vi "LaserFinding_Lines_v6.vi"(0 "Image In":T2, 7 "error in":errorcluster) -> (20 "Image Out":T2, 21 "Straight Edge (Find Vert. Edge)":T1 {"Point2 (Real-World)"."Y" format="%.2f"; "Point2 (Real-World)"."X" format="%.2f"; "Point1 (Real-World)"."Y" format="%.2f"; "Point1 (Real-World)"."X" format="%.2f"; "Point2 (Pixels)"."Y" format="%.2f"; "Point2 (Pixels)"."X" format="%.2f"; "Point1 (Pixels)"."Y" format="%.2f"; "Point1 (Pixels)"."X" format="%.2f"}, 22 "Straight Edge (Find Horiz. Edge)":T1 {"Point2 (Real-World)"."Y" format="%.2f"; "Point2 (Real-World)"."X" format="%.2f"; "Point1 (Real-World)"."Y" format="%.2f"; "Point1 (Real-World)"."X" format="%.2f"; "Point2 (Pixels)"."Y" format="%.2f"; "Point2 (Pixels)"."X" format="%.2f"; "Point1 (Pixels)"."Y" format="%.2f"; "Point1 (Pixels)"."X" format="%.2f"}, 27 "error out":errorcluster)   [LabVIEW 2014]
uses:
  <vilib>/vision/Image Controls.llb/IMAQ Image.ctl
  <vilib>/vision/Measure.llb/Edge Options.ctl
  <vilib>/vision/Measure.llb/Edge Polarity.ctl
  <vilib>/vision/Measure.llb/Straight Edge Options.ctl
  <vilib>/vision/Measure.llb/Straight Edge Process.ctl
  <vilib>/vision/NI_Vision_Development_Module.lvlib
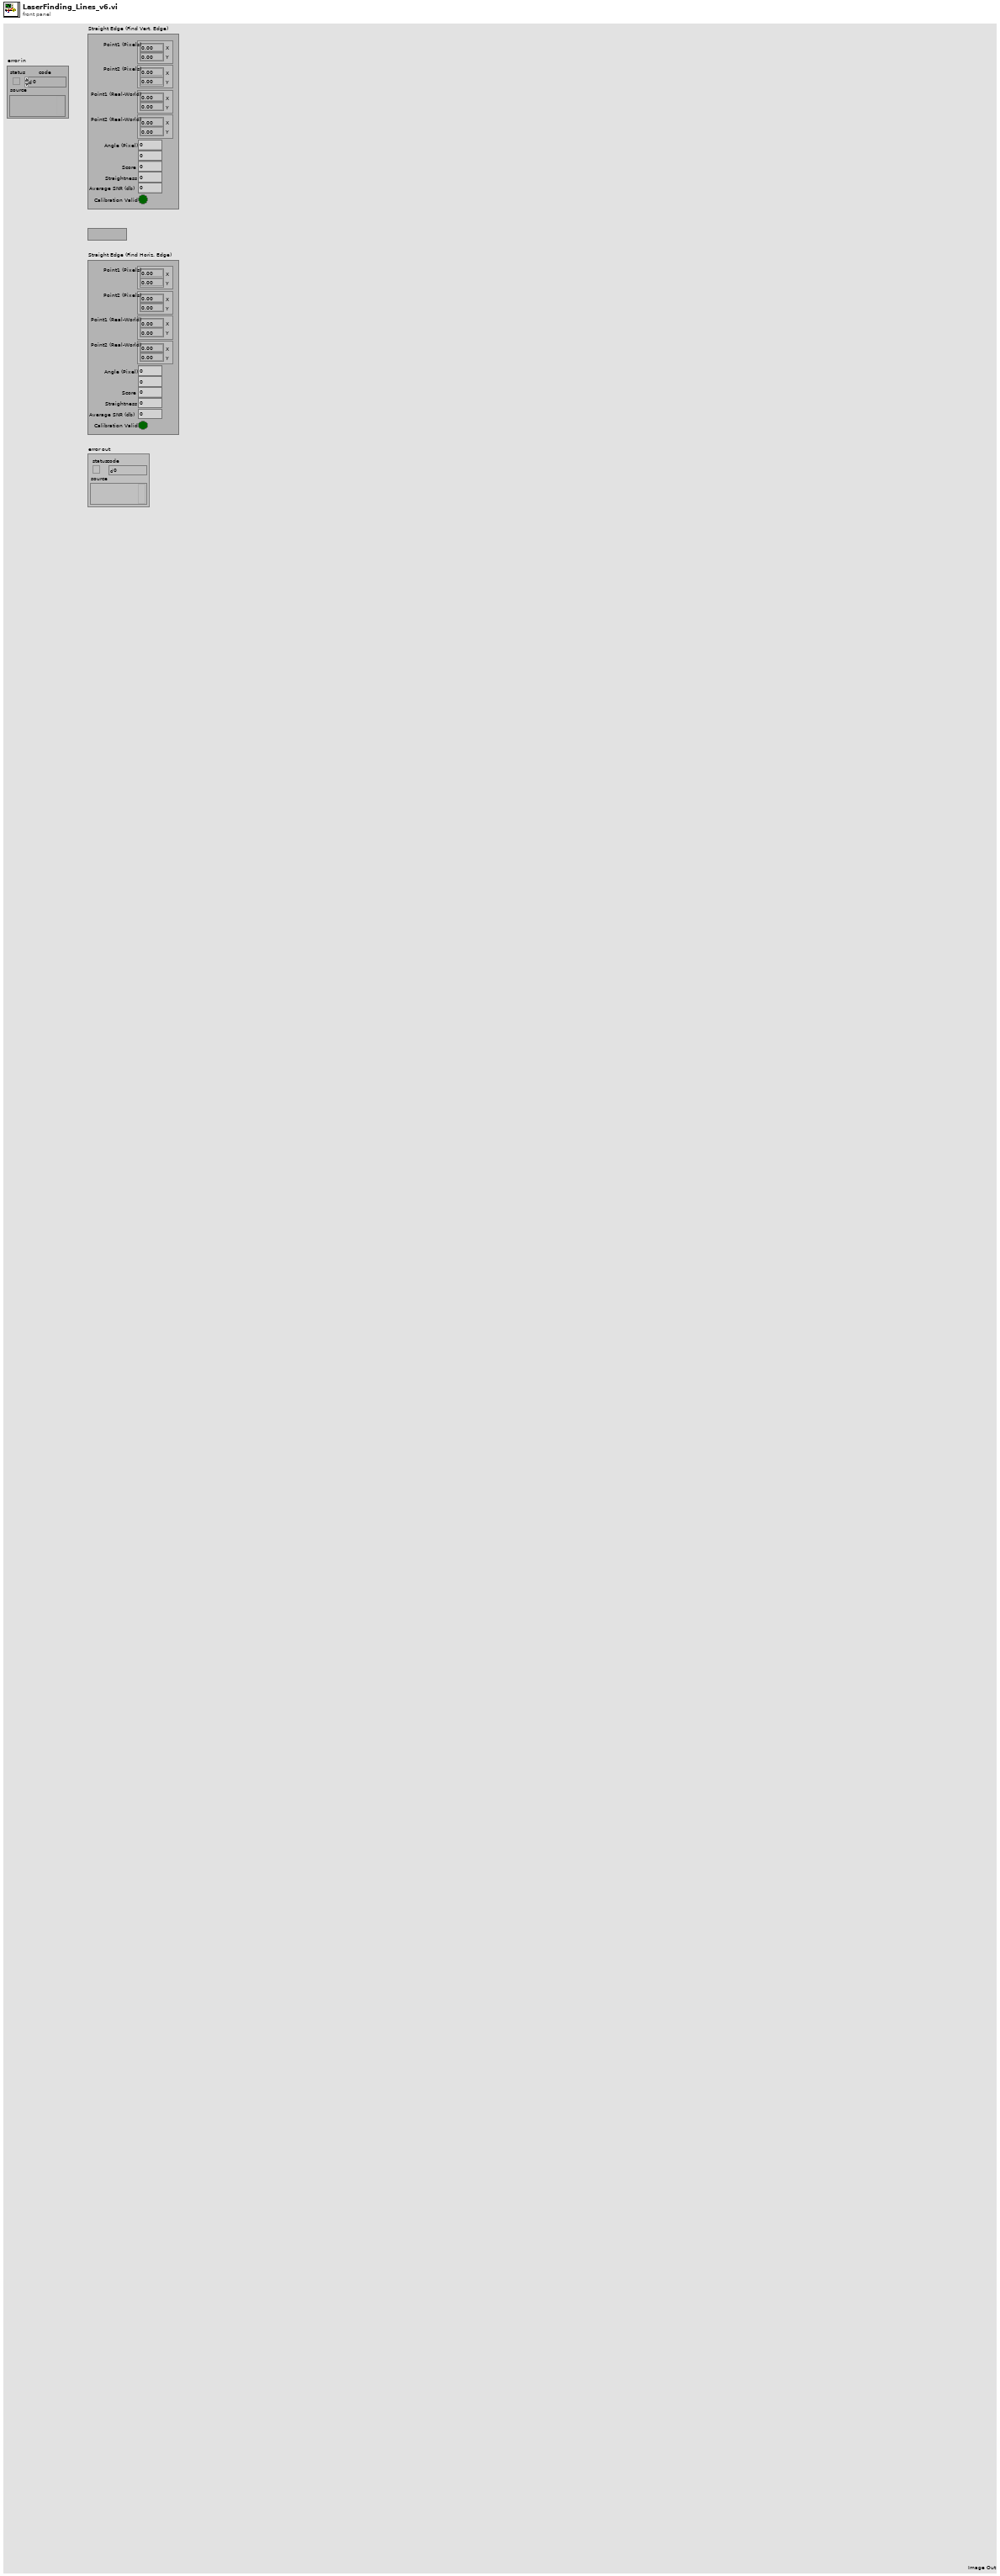
[diagram p1: front panel]
types:
  T1 = cluster{"Point1 (Pixels)":cluster{"X":sgl, "Y":sgl}, "Point2 (Pixels)":cluster{"X":sgl, "Y":sgl}, "Point1 (Real-World)":cluster{"X":sgl, "Y":sgl}, "Point2 (Real-World)":cluster{"X":sgl, "Y":sgl}, "Angle (Pixel)":dbl, "Angle (Real-World)":dbl, "Score":dbl, "Straightness":dbl, "Average SNR (db)":dbl, "Calibration Valid":bool}
  T2 = typedef "IMAQ Image.ctl" = refnum<image>
  T3 = typedef "Edge Options.ctl" = cluster{"Edge Polarity":T4, "Kernel Size":u32, "Width":u32, "Minimum Edge Strength":sgl, "Interpolation Type":enum32{"Zero Order", "Bilinear", "Quadratic", "Cubic", "Bilinear Fixed"}, "Data Processing Method":enum32{"Average", "Median"}}
  T4 = typedef "Edge Polarity.ctl" = u32
  T5 = cluster{"Search Direction":u32, "Edge Options":T3, "Show Search Area":bool, "Show Search Lines":bool, "Show Edges Found":bool, "Show Result":bool, "Search Area Color":u32, "Search Lines Color":u32, "Edge Locations Color":u32, "Result Color":u32, "Overlay Group Name":string}
  T6 = typedef "Straight Edge Options.ctl" = cluster{"Number of Lines":i32, "Type":T7, "Min. Score":dbl, "Max. Score":dbl, "Orientation":dbl, "Angle Range":dbl, "Angle Tolerance":dbl, "Step Size":u32, "Min. SNR (db)":dbl, "Min. Points (%)":dbl, "Hough Iterations":i32}
  T7 = typedef "Straight Edge Process.ctl" = enum32{"First Edge Rake", "Best Edge Rake", "Hough Edge Rake", "First Edge Projection", "Best Edge Projection"}
  T8 = cluster{"Global Rectangle":i32[], "Contours":cluster{"ID":enum32{"External", "Internal"}, "Type":u32, "Coordinates":i32[]}[]}
  T9 = cluster{"Measurement Parameter":i32, "Range Lower Value":dbl, "Range Upper Value":dbl, "Range":bool, "Measurement Type":bool}[]
  T10 = typedef "Image Type" = u32
  T11 = cluster{"histogram":u32[], "Minimal Value":sgl, "Maximal Value":sgl, "Starting Value":sgl, "Interval Width":sgl, "Mean Value":sgl, "Standard  Variation":sgl, "Area (pixels)":i32}
  T12 = cluster{"Point1 (Pixels)":cluster{"X":sgl, "Y":sgl}, "Point2 (Pixels)":cluster{"X":sgl, "Y":sgl}, "Point1 (Real-World)":cluster{"X":sgl, "Y":sgl}, "Point2 (Real-World)":cluster{"X":sgl, "Y":sgl}, "Angle (Pixel)":dbl, "Angle (Real-World)":dbl, "Score":dbl, "Straightness":dbl, "Average SNR (db)":dbl, "Calibration Valid":bool}[]
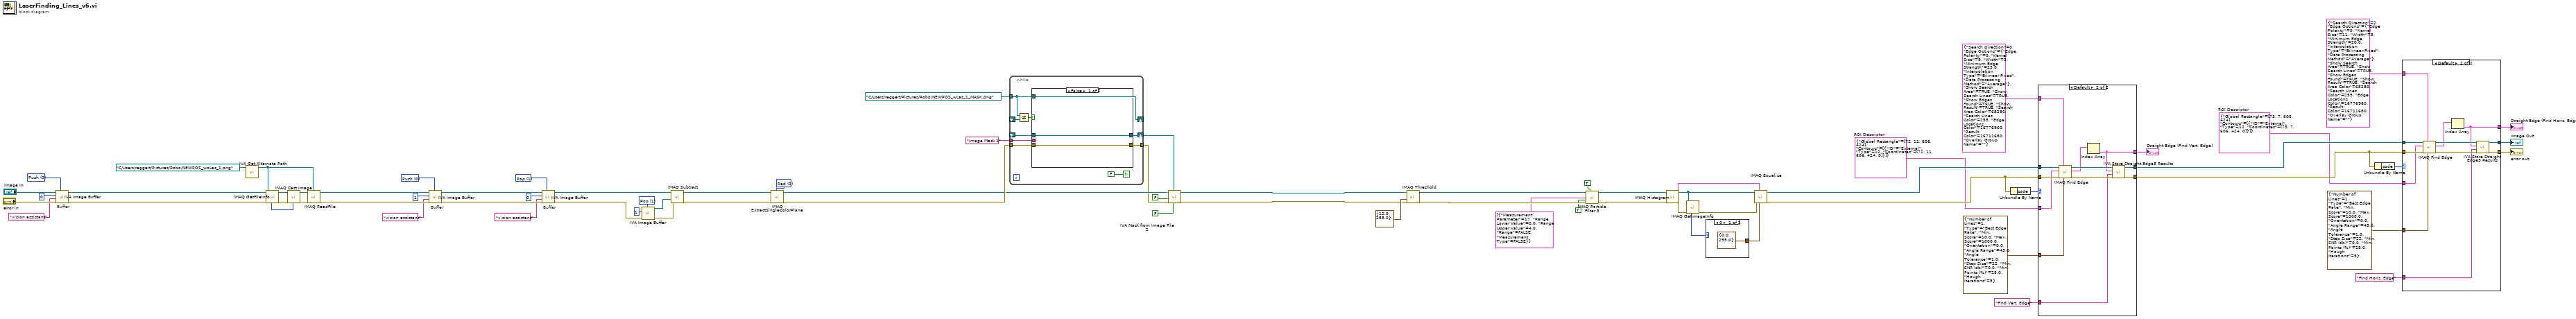
[diagram p0: block diagram]
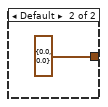
[diagram p4: hidden frame]
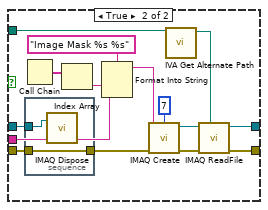
[diagram p5: hidden frame]
diagram:
  w10 = T8 {"Global Rectangle"=[73, 7, 606, 424], "Contours"=[{"ID"=enum."External", "Type"=12, "Coordinates"=[73, 7, 606, 424, 0]}]}  # ROI Descriptor
  w18 = T8 {"Global Rectangle"=[72, 11, 606, 424], "Contours"=[{"ID"=enum."External", "Type"=12, "Coordinates"=[72, 11, 606, 424, 0]}]}  # ROI Descriptor
  w43 = 0 items=["Red", "Green", "Blue", "Hue", "Saturation", "Luminance", "Value", "Intensity"] ("Color Plane")
  w49 = u16 1 items=["Push", "Pop", "Reset"] ("Function")
  w52 = u16 1 items=["Push", "Pop", "Reset"] ("Function")
  w57 = u16 0 items=["Push", "Pop", "Reset"] ("Function")
  w70 = u16 0 items=["Push", "Pop", "Reset"] ("Function")
  # "Buffer"
  # "Buffer"
  # "Buffer"
  n1 = call <vilib>:"IVA Image Buffer.vi"("Function"=w70, "error in (no error)"="error in", "Prefix"="vision assistant", "Buffer #"=0, "Image In"="Image In") -> ("error out"=w71:errorcluster, "Image Out"=w64:T2)  [unwired: 5 out]
  n2 = call <vilib>:"IVA Get Alternate Path.vi"("Path In"=path "C:/Users/reggert/Pictures/Robo/NEWPOS_woLas_1.png" ("File Path")) -> ("Path Out"=w60:path)  [unwired: 10 out]
  n3 = call "IMAQ GetFileInfo"("error in (no error)"=w71, "File Path"=w60) -> ("error out"=w66:errorcluster, "Image Type"=w62:T10)  [unwired: 8 out]
  n4 = call "IMAQ Cast Image"("Image Type"=w62, "error in (no error)"=w66, "Image Src"=w64) -> ("error out"=w65:errorcluster, "Image Dst Out"=w63:T2)  [unwired: 3 in, 4 out]
  n5 = call "IMAQ ReadFile"("File Path"=w60, "error in (no error)"=w65, "Image"=w63) -> ("error out"=w67:errorcluster, "Image Out"=w59:T2)  [unwired: 2 in, 5 out]
  n6 = call <vilib>:"IVA Image Buffer.vi"("Function"=w57, "error in (no error)"=w67, "Prefix"="vision assistant", "Buffer #"=1, "Image In"=w59) -> ("error out"=w58:errorcluster, "Image Out"=w54:T2)  [unwired: 5 out]
  n7 = call <vilib>:"IVA Image Buffer.vi"("Function"=w52, "error in (no error)"=w58, "Prefix"="vision assistant", "Buffer #"=0, "Image In"=w54) -> ("error out"=w53:errorcluster, "Image Out"=w45:T2)  [unwired: 5 out]
  n8 = call <vilib>:"IVA Image Buffer.vi"("Function"=w49, "error in (no error)"=w53, "Buffer #"=1) -> ("error out"=w46:errorcluster, "Image Out"=w47:T2)  [unwired: 2 in, 5 out]
  n9 = call "IMAQ Subtract"("Image Src A"=w45, "Image Src B"=w47, "error in (no error)"=w46) -> ("Image Dst Out"=w42:T2, "error out"=w44:errorcluster)  [unwired: 2 in, 2 out]
  n10 = call "IMAQ ExtractSingleColorPlane"("Color Plane"=w43, "error in (no error)"=w44, "Image Src"=w42) -> ("error out"=w41:errorcluster, "Image Dst Out"=w38:T2)  [unwired: 1 in, 6 out]
  n11 = while {
    shift-right: [w82] -> w35
    shift-left: _ -> [w81]
    tunnel: [w79] -> w36
    tunnel: w41 -> [w78]
    tunnel: path "C:/Users/reggert/Pictures/Robo/NEWPOS_wLas_1_MASK.png" ("FilePath") -> [w74]
    tunnel: "Image Mask 1" ("Step Name") -> [w77]
    shift-right: [w74] -> _
    shift-left: _ -> [w76]
    stop <- FALSE continue-if-true
    n12 = Not Equal?(x=w74, y=w76) -> (x != y?=w75:bool)
    n13 = case shown="False" w75 {
      tunnel: [w84 w96] -> w82
      tunnel: w81 -> [w84 w88]
      tunnel: [w83 w94] -> w79
      tunnel: w78 -> [w83 w89]
      tunnel: w74 -> [_ w86]
      tunnel: w77 -> [_ w90]
      frame False {
      }
      frame True {
        n14 = Call Chain() -> (call chain=w92:string[])
        n15 = stacked-sequence {
          tunnel: w89 -> [w100]
          tunnel: w88 -> [w101]
          tunnel: [w100] -> w87
          frame #0 {
            n16 = call "IMAQ Dispose"("Image"=w101) -> ()  [unwired: 2 in, 4 out]
          }
        }
        n17 = Index Array(array=w92) -> (element=w91:string)  [unwired: 1 in]
        n18 = Format Into String(format string="Image Mask %s %s" ("Image Name"), w91, w90) -> (resulting string=w99:string)  [unwired: 2 in, 1 out]
        n19 = call "IMAQ Create"("Border Size"=7, "Image Name"=w99, "error in (no error)"=w87) -> ("New Image"=w97:T2, "error out"=w95:errorcluster)  [unwired: 1 in, 1 out]
        n20 = call <vilib>:"IVA Get Alternate Path.vi"("Path In"=w86) -> ("Path Out"=w85:path)  [unwired: 10 out]
        n21 = call "IMAQ ReadFile"("File Path"=w85, "error in (no error)"=w95, "Image"=w97) -> ("error out"=w94:errorcluster, "Image Out"=w96:T2)  [unwired: 2 in, 5 out]
      }
    }
  }
  n22 = call <vilib>:"IVA Mask from Image File 2.vi"("Shrink"=FALSE, "Image Mask"=w35, "error in (no error)"=w36, "Out / In"=FALSE, "Image Src"=w38) -> ("error out"=w1:errorcluster, "Image Out"=w2:T2)  [unwired: 1 in, 4 out]
  n23 = call "IMAQ Threshold"("error in (no error)"=w1, "Range"=cluster{"Lower value":sgl, "Upper value":sgl} {"Lower value"=12.0, "Upper value"=255.0}, "Image Src"=w2) -> ("error out"=w32:errorcluster, "Image Dst Out"=w28:T2)  [unwired: 3 in, 4 out]
  n24 = call "IMAQ Particle Filter 3"("Image Src"=w28, "Connectivity 4/8 (8)"=TRUE, "Selection Values"=T9 [{"Measurement Parameter"=17, "Range Lower Value"=0.0, "Range Upper Value"=4.0, "Range"=FALSE, "Measurement Type"=FALSE}], "Keep/Remove Particles (F)"=TRUE ("Keep/Remove Particles"), "error in (no error)"=w32) -> ("Image Dst Out"=w23:T2, "error out"=w29:errorcluster)  [unwired: 4 in, 5 out]
  n25 = call "IMAQ Histogram"("error in (no error)"=w29, "Image"=w23) -> ("error out"=w22:errorcluster, "Histogram Report"=w25:T11)  [unwired: 3 in, 5 out]
  n26 = call "IMAQ GetImageInfo"("error in (no error)"=w22, "Image"=w23) -> ("error out"=w21:errorcluster, "Image Type"=w24:T10)  [unwired: 8 out]
  n27 = case shown="0" w24 {
    tunnel: [cluster{"Minimum":sgl, "Maximum":sgl} {"Minimum"=0.0, "Maximum"=255.0} ("Range") cluster{"Minimum":sgl, "Maximum":sgl} {"Minimum"=0.0, "Maximum"=0.0} ("Range")] -> w20
    frame 0 {
    }
    frame Default {
    }
  }
  n28 = call "IMAQ Equalize"("Range"=w20, "Histogram Report"=w25, "error in (no error)"=w21, "Image Src"=w23) -> ("error out"=w26:errorcluster, "Image Dst Out"=w19:T2)  [unwired: 2 in, 4 out]
  n29 = Unbundle By Name(w26) -> ("code"=w15:i32)
  n30 = case shown="Default" w15 {
    tunnel: w19 -> [w104 w116]
    tunnel: w26 -> [_ w115]
    tunnel: w18 -> [_ w109]
    tunnel: [w104 w113] -> w11
    tunnel: [_ w111] -> w17
    tunnel: "Find Vert. Edge" ("Step Name") -> [_ w110]
    tunnel: T6 {"Number of Lines"=1, "Type"=enum."Best Edge Rake", "Min. Score"=10.0, "Max. Score"=1000.0, "Orientation"=0.0, "Angle Range"=45.0, "Angle Tolerance"=1.0, "Step Size"=22, "Min. SNR (db)"=0.0, "Min. Points (%)"=25.0, "Hough Iterations"=5} ("Fit Options") -> [_ w108]
    tunnel: T5 {"Search Direction"=0, "Edge Options"={"Edge Polarity"=0, "Kernel Size"=9, "Width"=3, "Minimum Edge Strength"=23.0, "Interpolation Type"=enum."Bilinear Fixed", "Data Processing Method"=enum."Average"}, "Show Search Area"=TRUE, "Show Search Lines"=TRUE, "Show Edges Found"=TRUE, "Show Result"=TRUE, "Search Area Color"=65280, "Search Lines Color"=255, "Edge Locations Color"=16776960, "Result Color"=16711680, "Overlay Group Name"=""} ("Options") -> [_ w107]
    tunnel: [_ w105] -> w12
    frame -1074396199, -1074396198 {
      # "Discard Coordinate System Error"
    }
    frame Default {
      n31 = call "IMAQ Find Edge"("Line Fit Options"=w108, "Options"=w107, "error in (no error)"=w115, "ROI Descriptor"=w109, "Image"=w116) -> ("error out"=w112:errorcluster, "Straight Edges"=w106:T12, "Image Out"=w114:T2)  [unwired: 1 in, 3 out]
      n32 = Index Array(array=w106) -> (element=w105:T1)  [unwired: 1 in]
      n33 = call <vilib>:"IVA Store Straight Edge3 Results.vi"("error in (no error)"=w112, "Step Name"=w110, "Straight Edge"=w105, "Image in"=w114) -> ("error out"=w111:errorcluster, "Image dup"=w113:T2)  [unwired: 1 in, 5 out]
    }
  }
  "Straight Edge (Find Vert. Edge)" <- w12
  n34 = Unbundle By Name(w17) -> ("code"=w6:i32)
  n35 = case shown="Default" w6 {
    tunnel: w11 -> [w117 w129]
    tunnel: w17 -> [_ w128]
    tunnel: w10 -> [_ w122]
    tunnel: [w117 w126] -> w9
    tunnel: [_ w124] -> w8
    tunnel: "Find Horiz. Edge" ("Step Name") -> [_ w123]
    tunnel: T6 {"Number of Lines"=1, "Type"=enum."Best Edge Rake", "Min. Score"=10.0, "Max. Score"=1000.0, "Orientation"=0.0, "Angle Range"=45.0, "Angle Tolerance"=1.0, "Step Size"=22, "Min. SNR (db)"=0.0, "Min. Points (%)"=25.0, "Hough Iterations"=5} ("Fit Options") -> [_ w121]
    tunnel: T5 {"Search Direction"=2, "Edge Options"={"Edge Polarity"=0, "Kernel Size"=11, "Width"=3, "Minimum Edge Strength"=20.0, "Interpolation Type"=enum."Bilinear Fixed", "Data Processing Method"=enum."Average"}, "Show Search Area"=TRUE, "Show Search Lines"=TRUE, "Show Edges Found"=TRUE, "Show Result"=TRUE, "Search Area Color"=65280, "Search Lines Color"=255, "Edge Locations Color"=16776960, "Result Color"=16711680, "Overlay Group Name"=""} ("Options") -> [_ w120]
    tunnel: [_ w118] -> w3
    frame -1074396199, -1074396198 {
      # "Discard Coordinate System Error"
    }
    frame Default {
      n36 = call "IMAQ Find Edge"("Line Fit Options"=w121, "Options"=w120, "error in (no error)"=w128, "ROI Descriptor"=w122, "Image"=w129) -> ("error out"=w125:errorcluster, "Straight Edges"=w119:T12, "Image Out"=w127:T2)  [unwired: 1 in, 3 out]
      n37 = Index Array(array=w119) -> (element=w118:T1)  [unwired: 1 in]
      n38 = call <vilib>:"IVA Store Straight Edge3 Results.vi"("error in (no error)"=w125, "Step Name"=w123, "Straight Edge"=w118, "Image in"=w127) -> ("error out"=w124:errorcluster, "Image dup"=w126:T2)  [unwired: 1 in, 5 out]
    }
  }
  "Image Out" <- w9
  "error out" <- w8
  "Straight Edge (Find Horiz. Edge)" <- w3
